vi "Read XML.vi"() -> (0 "error out":errorcluster caption="错误输出", 3 "值":T1)   [LabVIEW 2016, in "Alarm interface.lvlib"]
uses:
  Alarm interface.lvlib
  <vilib>/Utility/xml.llb/Read From XML File(string).vi
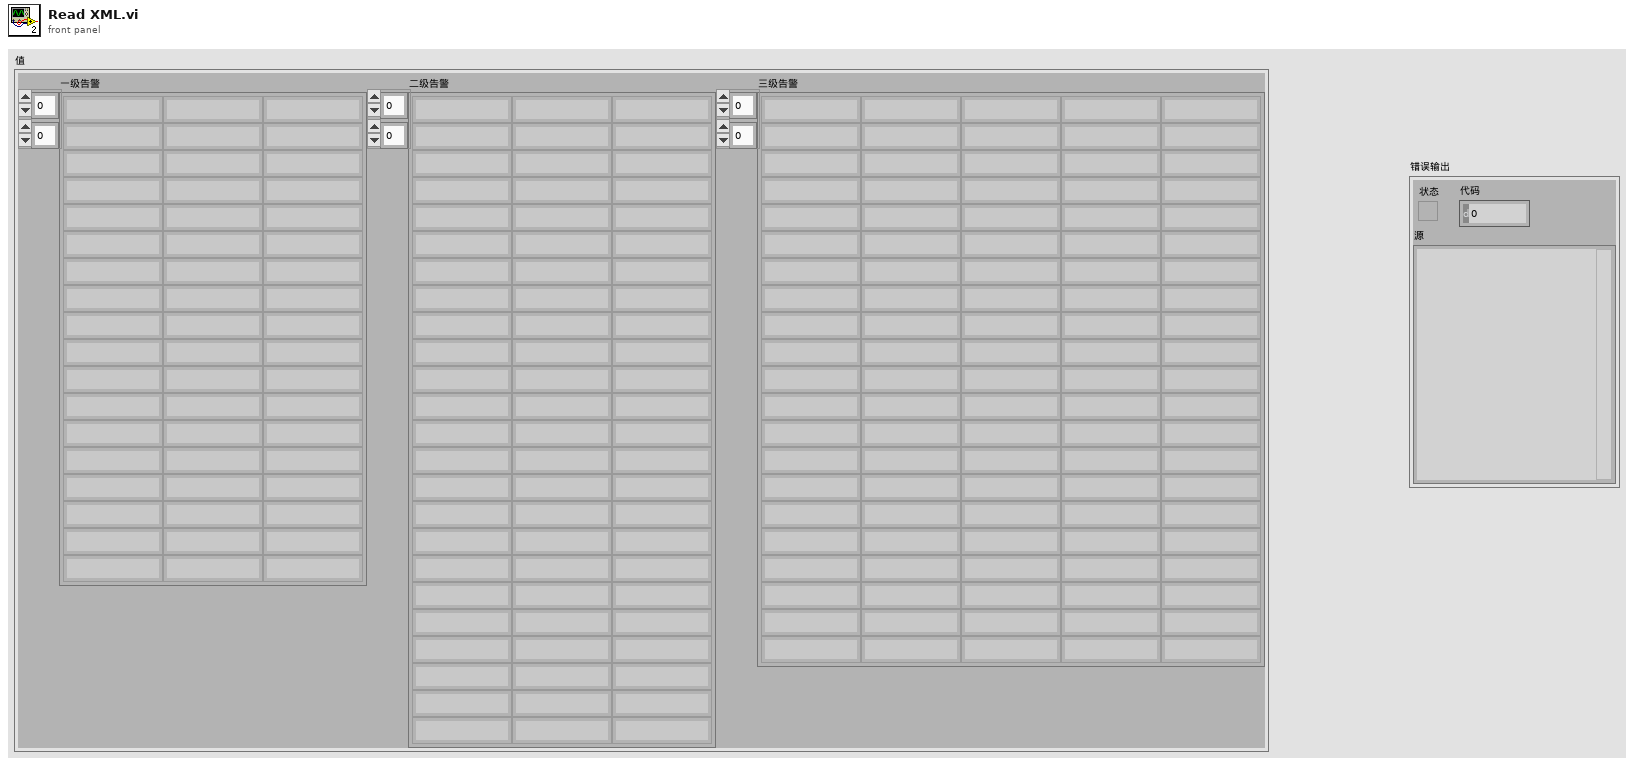
[diagram p1: front panel]
types:
  T1 = cluster{"一级告警":string[][], "二级告警":string[][], "三级告警":string[][]}
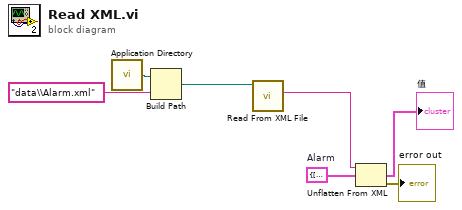
[diagram p0: block diagram]
diagram:
  w2 = T1 {"一级告警"=[], "二级告警"=[], "三级告警"=[]}  # Alarm
  n1 = call <vilib>:"Application Directory.vi"() -> ("Application Directory"=w5:path)
  n2 = Build Path(base path=w5, name or relative path="data\\Alarm.xml" ("名称或相对路径")) -> (appended path=w3:path)
  n3 = call-poly <vilib>:"Read From XML File.vi"("XML File Path"=w3) -> ("XML Elements"=w7:string)  [unwired: 8 in, 2 out]
  n4 = Unflatten From XML(xml string=w7, type=w2) -> (value=→"值":T1, error out=→"error out":errorcluster)  [unwired: 1 in]
